vi "Demo.vi"() -> ()   [LabVIEW 2020, in "File Tree.lvclass"]
uses:
  File Tree.lvclass
  File Tree.lvclass/File Tree.ctl
panel:
  out "Selected Tags":string[](array[string])
  in  "Tree":string[](tree)
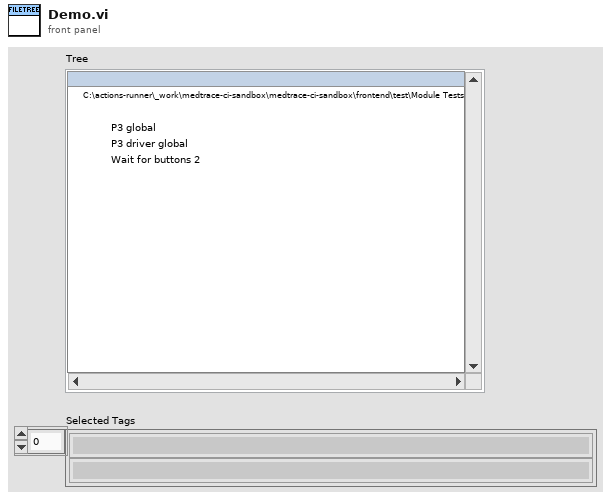
[diagram p1: front panel]
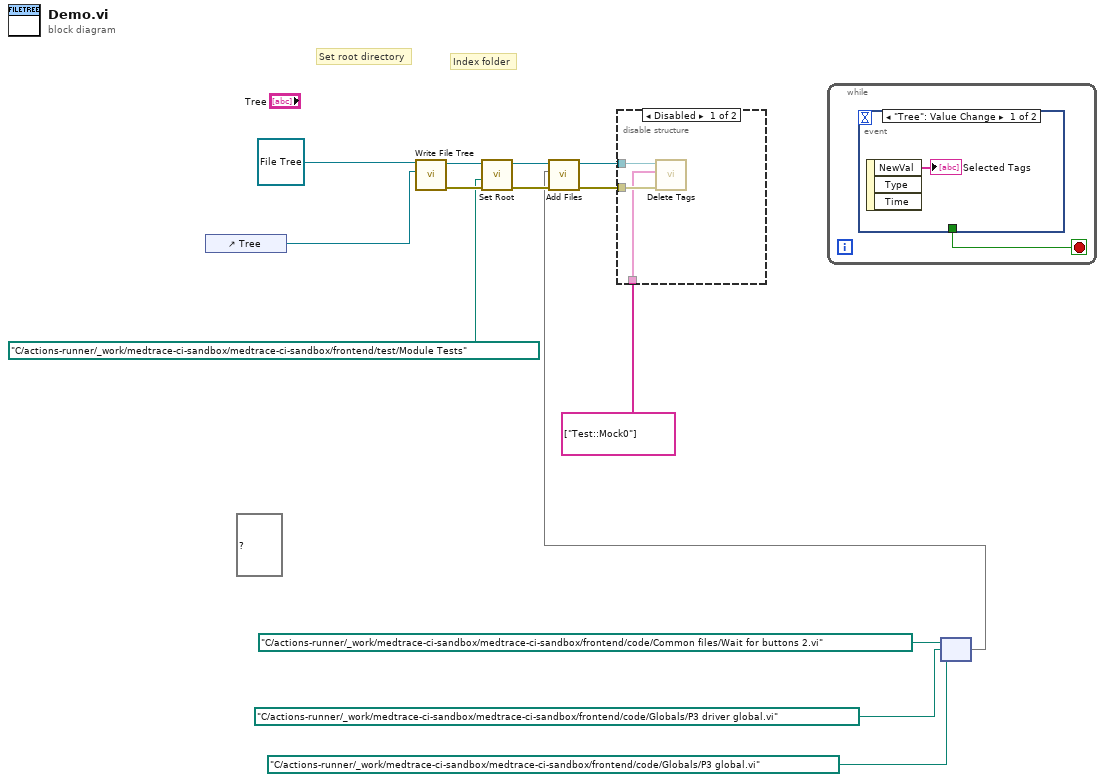
[diagram p0: block diagram]
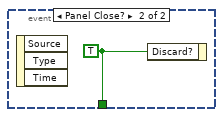
[diagram p2: hidden frame]
diagram:
  (unwired) set{path} {path "C:/git/astemes-lunit-coverage-report/source/Coverage Report/Commit to Include File.vi", path "C:/git/astemes-lunit-coverage-report/source/Coverage Report/Coverate Include File Path From Test Cases.vi", path "C:/git/astemes-lunit-coverage-report/source/Coverage Report/Create.vi", path "C:/git/astemes-lunit-coverage-report/source/Coverage Report/Generate XML File.vi", path "C:/git/astemes-lunit-coverage-report/source/Coverage Report/Load from Include File.vi", path "C:/git/astemes-lunit-coverage-report/source/Coverage Report/LUnit Configure.vi", path "C:/git/astemes-lunit-coverage-report/source/Coverage Report/LUnit Init.vi", path "C:/git/astemes-lunit-coverage-report/source/Coverage Report/LUnit Start Test.vi", path "C:/git/astemes-lunit-coverage-report/source/Coverage Report/LUnit Stop Test.vi", path "C:/git/astemes-lunit-coverage-report/source/Coverage Report/Recursive find VIs.vi", path "C:/git/astemes-lunit-coverage-report/source/Tree Helpers/File Tree/Add Files.vi", path "C:/git/astemes-lunit-coverage-report/source/Tree Helpers/File Tree/Delete Tags.vi", path "C:/git/astemes-lunit-coverage-report/source/Tree Helpers/File Tree/Demo.vi", path "C:/git/astemes-lunit-coverage-report/source/Tree Helpers/File Tree/Private/Find Common Path.vi", path "C:/git/astemes-lunit-coverage-report/source/Tree Helpers/File Tree/Set Root.vi", path "C:/git/astemes-lunit-coverage-report/source/Tree Helpers/File Tree/Write File Tree.vi"} ("VIs 2")
  # "Set root directory"
  # "Index folder"
  n1 = control-ref of="Tree"() -> (w13:refnum<vi>)
  n2 = call "Write File Tree.vi"("File Tree Reference"=w13, "File Tree In"=refnum<class "File Tree.lvclass"> refnum ("Support Utilities.lvlib:Tag Tree.lvclass")) -> ("error out"=w7:errorcluster, "File Tree Out"=w12:refnum<class "File Tree.lvclass">)  [unwired: 8 in]
  n3 = call "Set Root.vi"("error in (no error)"=w7, "Root Path"=path "C:/actions-runner/_work/medtrace-ci-sandbox/medtrace-ci-sandbox/frontend/test/Module Tests" ("VI Path"), "File Tree In"=w12) -> ("error out"=w6:errorcluster, "File Tree Out"=w8:refnum<class "File Tree.lvclass">)  [unwired: 7 in]
  n4 = while {
    stop <- w15 stop-if-true
    n5 = event shown="[0] \"Tree\": Value Change" {
      selector: _ -> [_ _]
      dyn-events: _ -> [_ _]
      timeout: _ -> [_ _]
      tunnel: [_ w17] -> w15
      event "Tree": Value Change {
        n6 = event-data() -> ("NewVal"=→"Selected Tags":string[])  [unwired: 1 in, 2 out]
      }
      event Panel Close? {
        w17 = TRUE ("Discard?")
        n7 = event-data() -> ()  [unwired: 1 in, 3 out]
        n8 = event-data ("Event Filter Node")("Discard?"=w17) -> ()  [unwired: 1 in, 1 out]
      }
    }
  }
  n9 = node(path "C:/actions-runner/_work/medtrace-ci-sandbox/medtrace-ci-sandbox/frontend/code/Common files/Wait for buttons 2.vi", path "C:/actions-runner/_work/medtrace-ci-sandbox/medtrace-ci-sandbox/frontend/code/Globals/P3 driver global.vi", path "C:/actions-runner/_work/medtrace-ci-sandbox/medtrace-ci-sandbox/frontend/code/Globals/P3 global.vi") -> (w1:set{path})
  n10 = call "Add Files.vi"("error in (no error)"=w6, "Files"=w1, "File Tree In"=w8) -> ("error out"=w10:errorcluster, "File Tree Out"=w11:refnum<class "File Tree.lvclass">)  [unwired: 7 in]
  n11 = disable-structure "Diagram Disable Structure" shown="Disabled" {
    disable-tunnel: w11 -> [w20 _]
    disable-tunnel: w10 -> [w19 _]
    disable-tunnel: string[] ["Test::Mock0"] ("Tag") -> [w18 _]
    frame Disabled {
      n12 = call "Delete Tags.vi"("error in (no error)"=w19, "Tag"=w18, "File Tree In"=w20) -> ()  [unwired: 7 in, 2 out]
    }
    frame Enabled {
    }
  }
